vi "FTW-Test-SQLite-JSON.vi"() -> (0 "Test Result":errorcluster)   [LabVIEW 2015]
uses:
  src/error/FTW-ERR-Assert-DeveloperError.vi
  src/error/FTW-ERR-StatusOK.vi
  src/error/FTW-ERR-ThrowError.vi
  src/error/FTW-ERR-ThrowInfo.vi
  src/error/FTW-ERR-CallChain.vi
  src/string/FTW-STR-ReplaceWhitespace.vi
  src/string/FTW-STR-Array-Delimit.vi
  src/error/FTW-ERR-Clear.vi
  src/regex/FTW-Regex-ReplaceAll.vi
  src/database/core/FTW-SQLite-Core-PrepareStatement.vi
  src/database/core/FTW-SQLite-Core-LibraryReturnValue.vi
  src/database/core/FTW-SQLite-Core-QueryDebug.vi
  codegen/xnode/FTW-SQLite-Fetch.xnode
  src/database/core/FTW-SQLite-Core-Structure.ctl
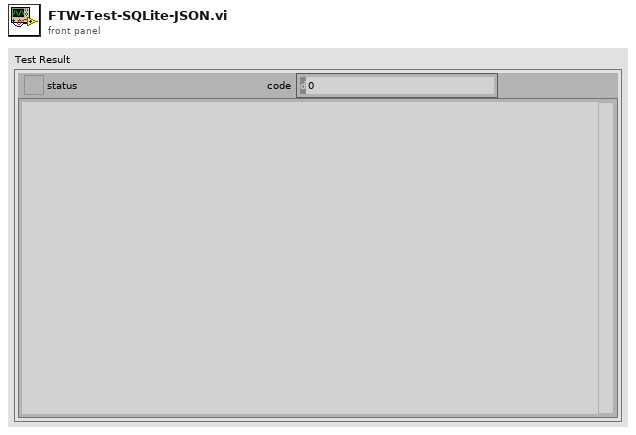
[diagram p1: front panel]
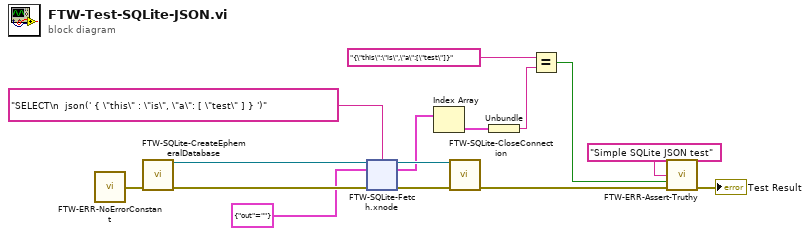
[diagram p0: block diagram]
diagram:
  n1 = call "FTW-ERR-NoErrorConstant.vi"() -> ("no error"=w15:errorcluster)
  n2 = call "FTW-SQLite-CreateEphemeralDatabase.vi"("error in"=w15) -> ("SQLite Connection"=w9:refnum<data-value>, "error out"=w6:errorcluster)  [unwired: 13 in]
  n3 = xnode "FTW-SQLite-Fetch.xnode"("SQLite Connection"=w9, "SQL Script"="SELECT\n  json(' { \"this\" : \"is\", \"a\": [ \"test\" ] } ')", "Row Datatype"=cluster{"out":string} {"out"=""}, "error in"=w6) -> ("SQLite Connection out"=w8:refnum<data-value>, "Result Set"=w3:cluster{"out":string}[], "error out"=w5:errorcluster)  [unwired: 1 out]
  n4 = Index Array(array=w3) -> (element=w14:cluster{"out":string})  [unwired: 1 in]
  n5 = call "FTW-SQLite-CloseConnection.vi"("SQLite Connection"=w8, "error in"=w5) -> ("error out"=w11:errorcluster)  [unwired: 13 in]
  n6 = Unbundle(w14) -> ("out"=w12:string)
  n7 = Equal?(x="{\"this\":\"is\",\"a\":[\"test\"]}", y=w12) -> (x = y?=w2:bool)
  n8 = call "FTW-ERR-Assert-Truthy.vi"("Assertion"="Simple SQLite JSON test", "Assertion holds true?"=w2, "error in"=w11) -> ("error out"=→"Test Result":errorcluster)  [unwired: 12 in]
